vi "WaitOn_Notifier.vi"(5 "Blackboard Group":string="Default", 6 "Ignore Previous_":bool, 7 "Notifier Name":string, 8 "Tag Root":string, 9 "Timeout (ms)":i32=-1, 10 "Message Type":variant, 11 "bt_Blackboard in":refnum<class "Blackboard.lvclass">) -> (0 "error out":errorcluster, 3 "Node Out":refnum<class "bt_Node.lvclass">)   [LabVIEW 2021, in "BT.lvlib"]
uses:
  BT.lvlib
  Blackboard/Blackboard.lvclass
  Support/Nodes/abs_Node/bt_Node.lvclass
  Support/Nodes/Leaves/Synch/Notifier/WaitOn/bt_WaitOn_Notifier.lvclass
  C:/Users/Tim/Documents/GitHub/LV_Behaviour_Tree/Source/Support/Nodes/Leaves/Synch/Parent/WaitOn/bt_WaitOn_Synch.lvclass
  C:/Users/Tim/Documents/GitHub/LV_Behaviour_Tree/Source/Support/Nodes/abs_Node/bt_Node.lvclass
  Support/Nodes/Leaves/Synch/Notifier/WaitOn/bt_WaitOn_Notifier.lvclass/bt_WaitOn_Notifier.ctl
  Support/Nodes/Leaves/Synch/Parent/WaitOn/bt_WaitOn_Synch.lvclass/bt_WaitOn_Synch.ctl
  Support/Nodes/Leaves/Synch/Notifier/WaitOn/Properties/Write Name.vi
  Support/Nodes/Leaves/Synch/Parent/WaitOn/Properties/Write Timeout.vi
  Support/Nodes/Leaves/Synch/Notifier/WaitOn/Properties/Write bt_Blackboard.vi
  Support/Nodes/Leaves/Synch/Notifier/WaitOn/Properties/Write Message Type.vi
  Support/Nodes/Leaves/Synch/Notifier/WaitOn/Properties/Write Tag Root.vi
  Support/Nodes/Leaves/Synch/Notifier/WaitOn/Properties/Write Blackboard Group.vi
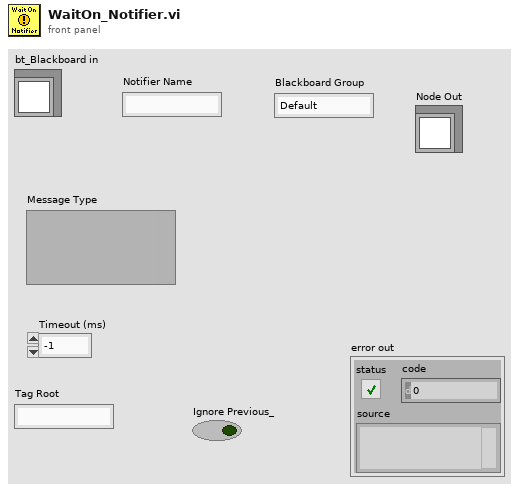
[diagram p1: front panel]
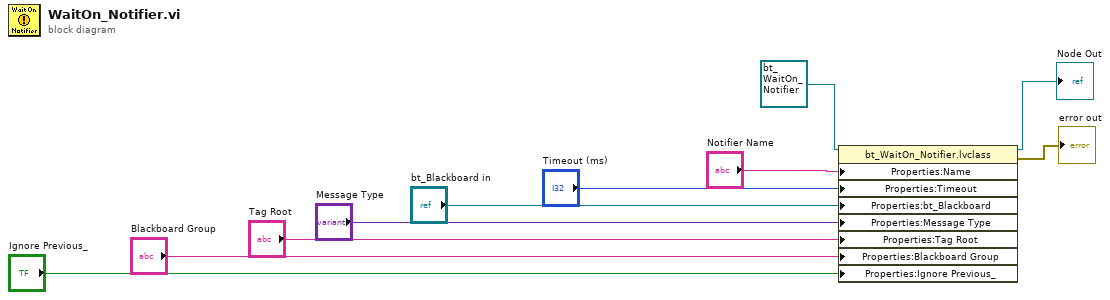
[diagram p0: block diagram]
diagram:
  n1 = property class="bt_WaitOn_Notifier.lvclass"(reference=refnum<class "bt_WaitOn_Notifier.lvclass"> refnum ("BT.lvlib:bt_WaitOn_Notifier.lvclass"), "Properties:Name"="Notifier Name", "Properties:Timeout"="Timeout (ms)", "Properties:bt_Blackboard"="bt_Blackboard in", "Properties:Message Type"="Message Type", "Properties:Tag Root"="Tag Root", "Properties:Blackboard Group"="Blackboard Group", "Properties:Ignore Previous_"="Ignore Previous_") -> (reference out=→"Node Out":refnum<class "bt_WaitOn_Notifier.lvclass">, error out=→"error out":errorcluster)  [unwired: 1 in]
